vi "Available AI.vi"(8 "error in (no error)":errorcluster, 11 "VisaComms in":refnum<class "VisaComms.lvclass">) -> (0 "error out":errorcluster, 2 "Available AI":T1[](array[typedef]), 3 "VisaComms out":refnum<class "VisaComms.lvclass">)   [LabVIEW 2020, in "CTI.lvlib" / "VisaComms.lvclass"]
uses:
  VisaComms.lvclass
  Available AI.ctl
  ADC Number.ctl
  GPIO Number.ctl
  VisaComms.lvclass/VisaComms.ctl
  CTI.lvlib
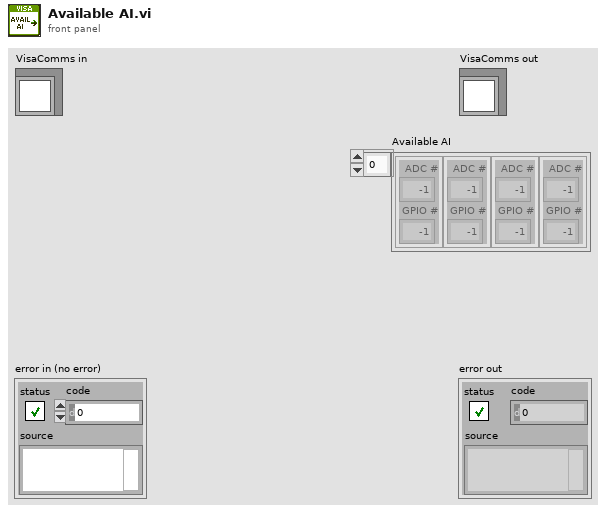
[diagram p1: front panel]
types:
  T1 = typedef "CTI.lvlib/Available AI.ctl" = cluster{"ADC #":T2, "GPIO #":T3}
  T2 = typedef "CTI.lvlib/ADC Number.ctl" = i8
  T3 = typedef "CTI.lvlib/GPIO Number.ctl" = i8
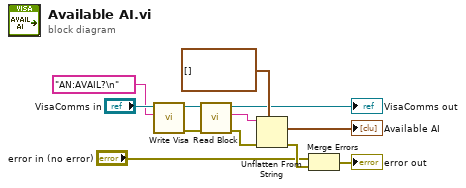
[diagram p0: block diagram]
diagram:
  n1 = call "Write Visa.vi"("write buffer"="AN:AVAIL?\n", "VisaComms in"="VisaComms in") -> ("error out"=w8:errorcluster, "VisaComms out"=w9:refnum<class "VisaComms.lvclass">)  [unwired: 7 in, 1 out]
  n2 = call "Read Block.vi"("error in (no error)"=w8, "VisaComms in"=w9) -> ("error out"=w12:errorcluster, "Block"=w7:string, "VisaComms out"=→"VisaComms out":refnum<class "VisaComms.lvclass">)  [unwired: 7 in]
  n3 = Unflatten From String(type=T1[] [] ("Available AI"), binary string=w7, error in (no error)=w12) -> (value=→"Available AI":T1[], error out=w3:errorcluster)  [unwired: 2 in, 1 out]
  n4 = Merge Errors("error in (no error)", w3) -> (→"error out":errorcluster)
